vi "Close File.vi"(8 "error in (no error)":errorcluster, 11 "Text File in":refnum<class "Text File.lvclass">) -> (0 "error out":errorcluster, 3 "Text File out":refnum<class "Text File.lvclass">)   [LabVIEW 2018, in "MVA Framework.lvlib" / "Text File.lvclass"]
uses:
  Text File.lvclass
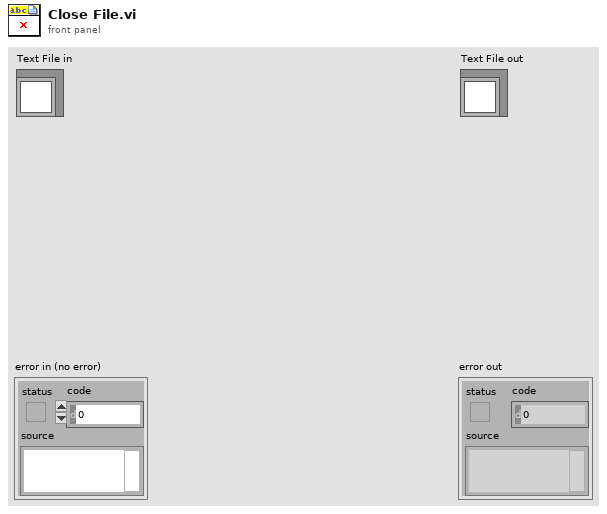
[diagram p1: front panel]
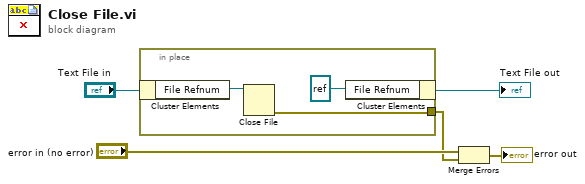
[diagram p0: block diagram]
diagram:
  n1 = in-place {
    in-place-border: [w6] -> w2
    n2 = in-place-cluster #1("Text File in") -> ("File Refnum"=w7:refnum<file>)
    n3 = Close File(refnum=w7) -> (error out=w6:errorcluster)  [unwired: 1 in, 1 out]
    n4 = in-place-cluster #1("File Refnum"=refnum<file> refnum) -> (→"Text File out":refnum<class "Text File.lvclass">)
  }
  n5 = Merge Errors("error in (no error)", w2) -> (→"error out":errorcluster)
